vi "run.get_from_asset.vi"(8 "error in":errorcluster, 10 "asset":refnum<class "asset.lvclass">, 11 "Nominal Client in":refnum<class "Nominal Client.lvclass">) -> (0 "error out":errorcluster, 2 "Run":refnum<class "Run.lvclass">[](array[class]), 3 "Nominal Client out":refnum<class "Nominal Client.lvclass">)   [LabVIEW 2020]
doc: "Fetches the runs with the given asset"
uses:
  Nominal Client.lvclass
  Run/Run.lvclass
  asset/asset.lvclass
  <vilib>/JDP Science/JSONtext/Next JSON Value.vi
  <vilib>/JDP Science/JSONtext/String Subset.vi
  <vilib>/JDP Science/JSONtext/Parsing/Advance past next JSON Value (inlined COPY).vi
  <vilib>/JDP Science/JSONtext/Parsing/Advance past whitespace.vi
  <vilib>/JDP Science/JSONtext/Parsing/Advance past String.vi
  <vilib>/JDP Science/JSONtext/Parsing/Advance past Number.vi
  <vilib>/JDP Science/JSONtext/Parsing/Advance past Line Ending.vi
  <vilib>/JDP Science/JSONtext/Parsing/Parse Full Path or Item Name.vi
  <vilib>/JDP Science/JSONtext/Parsing/Advance past Array.vi
  <vilib>/JDP Science/JSONtext/Parsing/Advance past Object.vi
  <vilib>/JDP Science/JSONtext/support/Error Cluster From Code.vi
  <vilib>/JDP Science/JSONtext/Offset/Find Item Locations by Path.vi
  Nominal Client.lvclass/Nominal Client.ctl
  <vilib>/JDP Science/JSONtext/JSONtext.lvlib
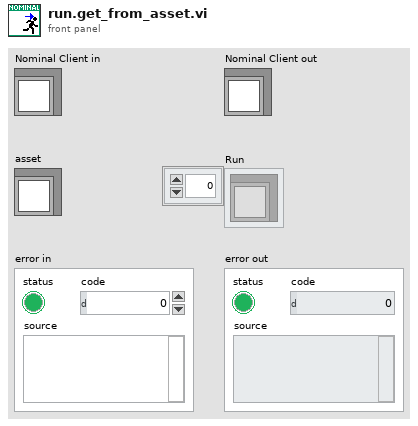
[diagram p1: front panel]
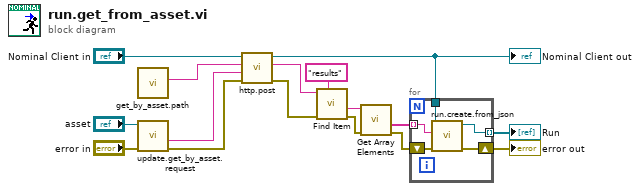
[diagram p0: block diagram]
diagram:
  n1 = call "get_by_asset.path.vi"() -> ("path"=w12:string)  [unwired: 11 in]
  n2 = call "update.get_by_asset.request.vi"("error in"="error in", "asset"="asset") -> ("error out"=w13:errorcluster, "Request"=w14:string)  [unwired: 8 in]
  n3 = call "http.post.vi"("error in"=w13, "Request body"=w14, "Path"=w12, "Nominal Client in"="Nominal Client in") -> ("error out"=w4:errorcluster, "Response"=w3:string, "Nominal Client out"=w1:refnum<class "Nominal Client.lvclass">)  [unwired: 4 in, 1 out]
  "Nominal Client out" <- w1
  n4 = call <vilib>:"Find Item.vi"("$Path or Item Name"="results", "error in (no error)"=w4, "JSON"=w3) -> ("error out"=w5:errorcluster, "<JSON>"=w2:string)  [unwired: 5 in, 2 out]
  n5 = call <vilib>:"Get Array Elements.vi"("error in (no error)"=w5, "JSON"=w2) -> ("error out"=w6:errorcluster, "<JSON>"=w7:string[])  [unwired: 7 in, 1 out]
  n6 = for {
    tunnel: [w21] -> w16 mode=indexing
    tunnel: w7 -> [w19] mode=indexing
    shift-right: [w20] -> w15
    shift-left: w6 -> [w18]
    tunnel: w1 -> [w17]
    n7 = call "run.create.from_json.vi"("error in"=w18, "JSON"=w19, "Nominal Client"=w17) -> ("error out"=w20:errorcluster, "Run out"=w21:refnum<class "Run.lvclass">)  [unwired: 7 in]
  }
  "error out" <- w15
  "Run" <- w16
